vi "Check if Cell if Ref to Sheet.vi"(11 "Value":variant) -> (2 "Sheet Name":string, 3 "Sheet Ref":bool)   [LabVIEW 2025, in "Config from Excel Table.lvclass"]
uses:
  Config from Excel Table.lvclass
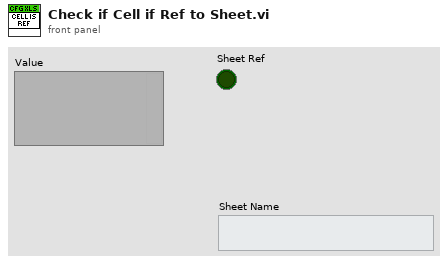
[diagram p1: front panel]
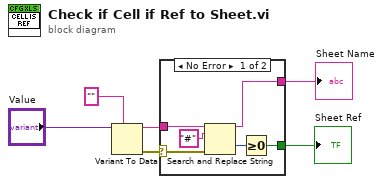
[diagram p0: block diagram]
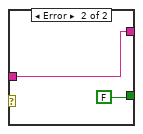
[diagram p2: hidden frame]
diagram:
  n1 = Variant To Data(type="", Variant="Value") -> (data=w2:string, error out=w6:errorcluster)  [unwired: 1 in]
  n2 = case shown="No Error" w6 {
    selector: w6 -> [w10 _]
    tunnel: [w9 FALSE] -> w3
    tunnel: w2 -> [w8 w13]
    tunnel: [w7 w13] -> w1
    frame No Error {
      n3 = Search and Replace String(input string=w8, search string="#", error in=w10) -> (result string=w7:string, offset past replacement=w12:i32)  [unwired: 5 in, 2 out]
      n4 = Greater Or Equal To 0?(x=w12) -> (x >= 0?=w9:bool)
    }
    frame Error {
    }
  }
  "Sheet Ref" <- w3
  "Sheet Name" <- w1
